vi "SRAD Create 32f.vi"(8 "Error In":errorcluster, 9 "Dimensions":T6={"Depth"=1, "Height"=1, "Width"=1} {"Width" min=1; "Height" min=1; "Depth" min=1}, 11 "Device In":T2) -> (0 "Error Out":errorcluster, 3 "SRAD Filter Object":T1={"Device In"=0, "Program Handle"=0, "N"={"Device ID"=0, "Memeroy ID"=0, "Dimension"={"Depth"=0, "Height"=0, "Width"=0}, "Memory Type"=enum."32f"}, "N + 1"={"Device ID"=0, "Memeroy ID"=0, "Dimension"={"Depth"=0, "Height"=0, "Width"=0}, "Memory Type"=enum."32f"}, "Dimensions"={"Depth"=1, "Height"=1, "Width"=1}, "Diffusivity"={"Device ID"=0, "Memeroy ID"=0, "Dimension"={"Depth"=0, "Height"=0, "Width"=0}, "Memory Type"=enum."32f"}} {"Diffusivity"."Dimension"."Width" min=1; "Diffusivity"."Dimension"."Height" min=1; "Diffusivity"."Dimension"."Depth" min=1; "Dimensions"."Width" min=1; "Dimensions"."Height" min=1; "Dimensions"."Depth" min=1; "N + 1"."Dimension"."Width" min=1; "N + 1"."Dimension"."Height" min=1; "N + 1"."Dimension"."Depth" min=1; "N"."Dimension"."Width" min=1; "N"."Dimension"."Height" min=1; "N"."Dimension"."Depth" min=1})   [LabVIEW 2012, in "OpenCLV x64.lvlib"]
uses:
  OpenCLV x64.lvlib
  Controls/Device ID.ctl
  User Controls/Array Dimensions.ctl
  Controls/SRAD Filter Object.ctl
  Controls/Program Handle.ctl
  Controls/Memory Object.ctl
  Controls/Memory ID.ctl
  Controls/Memory Type.ctl
  Allocate Memory/AllocateMemory_32f.vi
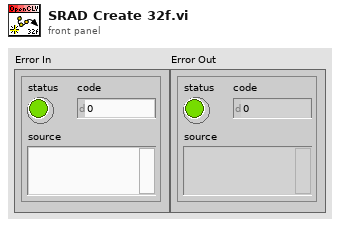
[diagram p1: front panel]
types:
  T1 = typedef "OpenCLV x64.lvlib/SRAD Filter Object.ctl" = cluster{"Device In":T2, "Program Handle":T3, "N":T4, "N + 1":T4, "Dimensions":T6, "Diffusivity":T4}
  T2 = typedef "OpenCLV x64.lvlib/Device ID.ctl" = u64
  T3 = typedef "OpenCLV x64.lvlib/Program Handle.ctl" = u64
  T4 = typedef "OpenCLV x64.lvlib/Memory Object.ctl" = cluster{"Device ID":T2, "Memeroy ID":T5, "Dimension":T6, "Memory Type":T7}
  T5 = typedef "OpenCLV x64.lvlib/Memory ID.ctl" = u64
  T6 = typedef "Array Dimensions.ctl" = cluster{"Depth":u64, "Height":u64, "Width":u64}
  T7 = typedef "OpenCLV x64.lvlib/Memory Type.ctl" = enum16{"32f", "u8", "i8", "u16", "i16", "u32", "i32", "64f"}
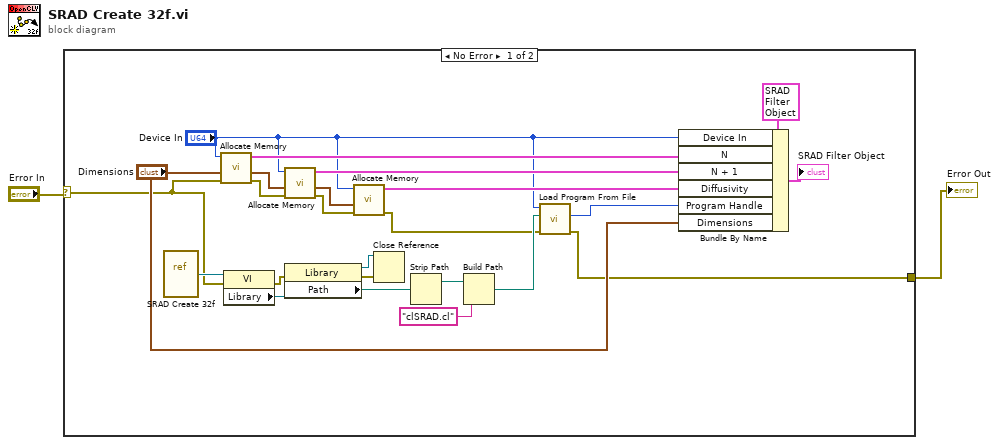
[diagram p0: block diagram]
diagram:
  n1 = case shown="No Error" "Error In" {
    selector: "Error In" -> [w3 w27]
    tunnel: [w7 w27] -> w1
    frame No Error {
      n2 = vi-ref "SRAD Create 32f.vi"() -> (w22:refnum<vi>)
      n3 = call-poly "Allocate Memory.vi"("Error In"=w3, "Dimension"="Dimensions", "Device In"="Device In") -> ("Error Out"=w20:errorcluster, "Dimension Out"=w19:T6, "Memory Object"=w16:T4)  [unwired: 6 in]
      n4 = property class="VI"(reference=w22, error in=w3) -> (error out=w4:errorcluster, "Library"=w24:refnum<vi>)  [unwired: 1 out]
      n5 = call-poly "Allocate Memory.vi"("Error In"=w20, "Dimension"=w19, "Device In"="Device In") -> ("Error Out"=w12:errorcluster, "Dimension Out"=w11:T6, "Memory Object"=w15:T4)  [unwired: 6 in]
      n6 = property class="Library"(reference=w24, error in=w4) -> (reference out=w5:refnum<vi>, error out=w6:errorcluster, "Path"=w23:path)
      n7 = call-poly "Allocate Memory.vi"("Error In"=w12, "Dimension"=w11, "Device In"="Device In") -> ("Error Out"=w9:errorcluster, "Memory Object"=w10:T4)  [unwired: 6 in, 1 out]
      n8 = Close Reference(reference=w5, error in (no error)=w6) -> ()  [unwired: 1 out]
      n9 = Strip Path(path=w23) -> (stripped path=w26:path)  [unwired: 1 out]
      n10 = Build Path(base path=w26, name or relative path="clSRAD.cl") -> (appended path=w21:path)
      n11 = call "Load Program From File.vi"("Error In"=w9, "Program Path"=w21, "Device In"="Device In") -> ("Error Out"=w7:errorcluster, "Program Handle"=w13:T3)  [unwired: 6 in, 1 out]
      n12 = Bundle By Name(cluster=T1 {"Device In"=0, "Program Handle"=0, "N"={"Device ID"=0, "Memeroy ID"=0, "Dimension"={"Depth"=0, "Height"=0, "Width"=0}, "Memory Type"=enum."32f"}, "N + 1"={"Device ID"=0, "Memeroy ID"=0, "Dimension"={"Depth"=0, "Height"=0, "Width"=0}, "Memory Type"=enum."32f"}, "Dimensions"={"Depth"=0, "Height"=0, "Width"=0}, "Diffusivity"={"Device ID"=0, "Memeroy ID"=0, "Dimension"={"Depth"=0, "Height"=0, "Width"=0}, "Memory Type"=enum."32f"}} ("Anisotropic Filter Object"), "Device In"="Device In", "N"=w16, "N + 1"=w15, "Diffusivity"=w10, "Program Handle"=w13, "Dimensions"="Dimensions") -> (→"SRAD Filter Object":T1)
    }
    frame Error {
    }
  }
  "Error Out" <- w1
